vi "SendCommandToDeviceTCPWithRetry.vi"(6 "timeout ms":i32=100, 7 "ms to wait between retries":u32=50, 8 "error in":errorcluster, 9 "str command":string, 10 "connection refnum in":refnum<k5>, 11 "IP address":string) -> (0 "error out":errorcluster, 1 "str out":string, 2 "str to byte array":u8[](array[numeric]), 3 "connection refnum out":refnum<k5>)   [LabVIEW 2023]
doc: "Send a string command using a TCP connection.\nRetry multiple times until a connection is successful."
uses:
  GlobalVarsNetwork.vi
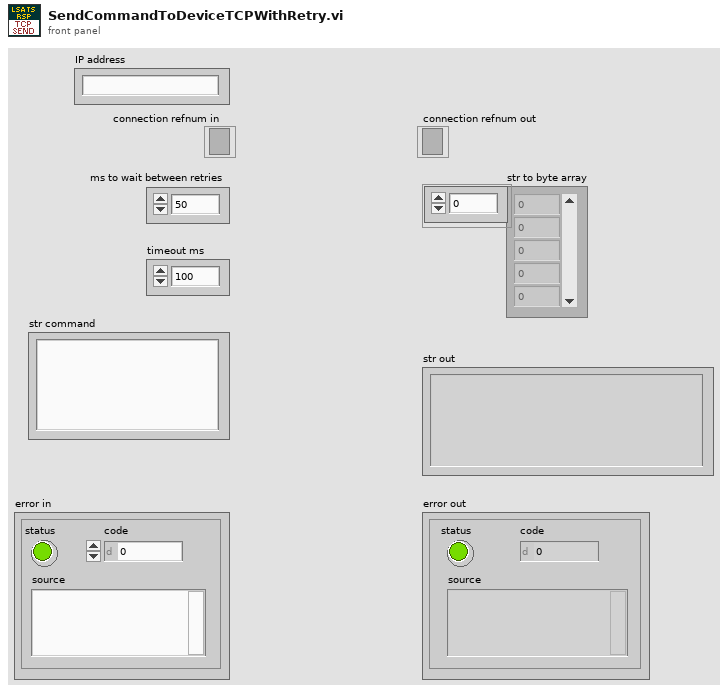
[diagram p1: front panel]
types:
  T1 = enum16{"Standard", "Buffered", "CRLF", "Immediate"}
  T2 = cluster{"XY_IP_ADDRESS":string, "Z_IP_ADDRESS":string, "Port":u16, "connection refnum x,y":refnum<k5>, "connection refnum z":refnum<k5>}
  T3 = enum16{"Initial Success", "Retry Successful", "Retry Failed"}
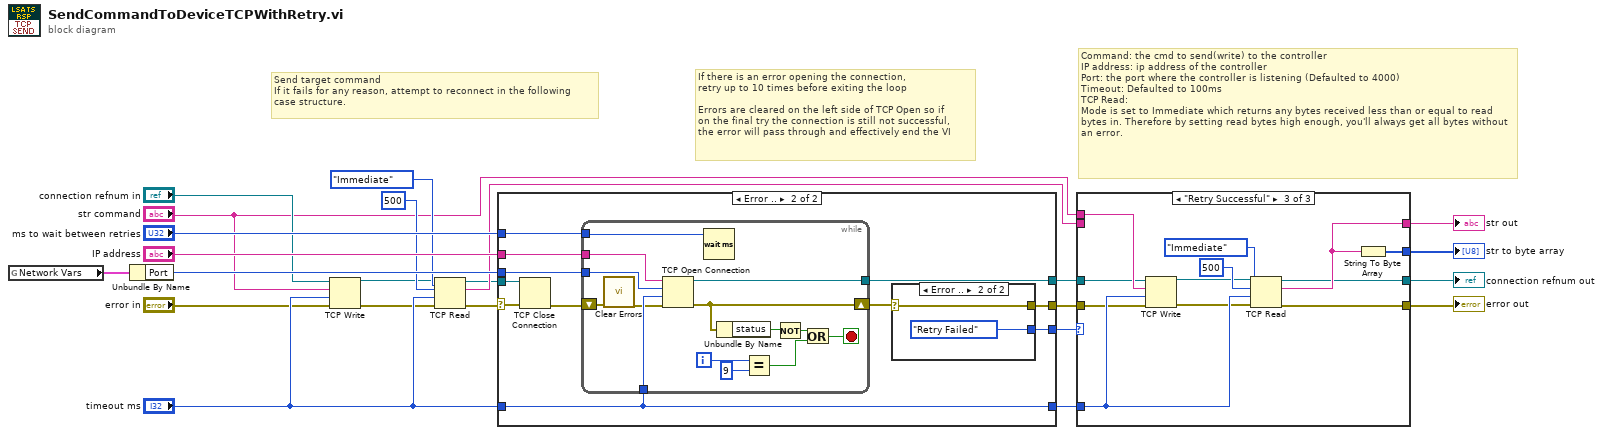
[diagram p0: block diagram]
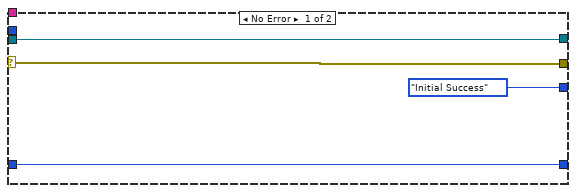
[diagram p2: hidden frame]
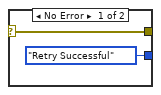
[diagram p3: hidden frame]
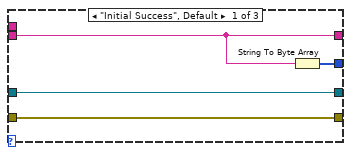
[diagram p4: hidden frame]
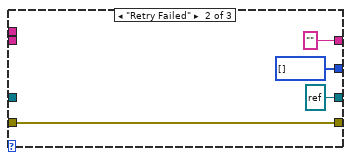
[diagram p5: hidden frame]
diagram:
  # "Send target command\nIf it fails for any reason, attempt to reconnect in the following\ncase structure."
  # "If there is an error opening the connection,\nretry up to 10 times before exiting the loop\n\nErrors are cleared on the left side of TCP Open so if \non the final try the connection is still not successful, \nthe error will pass through and effectively end the VI"
  # "Command: the cmd to send(write) to the controller\nIP address: ip address of the controller\nPort: the port where the controller is listening (Defaulted to 4000)\nTimeout: Defaulted to 100ms\nTCP Read:\nMode is set to Immediate which returns any bytes received less than or equal to read bytes in. Therefore by setting read bytes high enough, you'll always get all bytes without an error."
  n1 = global read "GlobalVarsNetwork.vi" "Network Vars"() -> (w20:T2)
  n2 = Unbundle By Name(w20) -> ("Port"=w19:u16)
  n3 = TCP Write(connection ID="connection refnum in", data in="str command", error in (no error)="error in", 9:"timeout ms") -> (connection ID out=w11:refnum<k5>, error out=w10:errorcluster)  [unwired: 1 out]
  n4 = TCP Read(connection ID=w11, bytes to read=500, error in (no error)=w10, 7:T1."Immediate" ("mode (standard)"), 9:"timeout ms") -> (connection ID out=w1:refnum<k5>, data out=w5:string, error out=w2:errorcluster)
  n5 = case shown="Error .." w2 {
    selector: w2 -> [w24 w29]
    tunnel: w19 -> [_ w38]
    tunnel: [w27 w37] -> w18
    tunnel: "ms to wait between retries" -> [_ w36]
    tunnel: "IP address" -> [_ w35]
    tunnel: "timeout ms" -> [w26 w34]
    tunnel: w1 -> [w27 w30]
    tunnel: [w26 w34] -> w7
    tunnel: [T3."Initial Success" w32] -> w4
    tunnel: [w24 w31] -> w3
    frame No Error {
    }
    frame Error {
      n6 = TCP Close Connection(connection ID=w30, error in (no error)=w29) -> (error out=w28:errorcluster)  [unwired: 1 in, 1 out]
      n7 = while {
        tunnel: w35 -> [w56]
        tunnel: w38 -> [w55]
        tunnel: [w54] -> w37
        tunnel: w34 -> [w47]
        shift-right: [w48] -> w33
        shift-left: w28 -> [w46]
        tunnel: w36 -> [w44]
        i -> [w53]
        stop <- w43 stop-if-true
        n8 = call <vilib>:"Clear Errors.vi"("error in (no error)"=w46) -> ("error out"=w45:errorcluster)  [unwired: 5 in, 1 out]
        n9 = TCP Open Connection(address=w56, remote port or service name=w55, timeout ms (60000)=w47, error in (no error)=w45) -> (connection ID=w54:refnum<k5>, error out=w48:errorcluster)  [unwired: 1 in]
        n10 = Wait (ms)(milliseconds to wait=w44) -> ()  [unwired: 1 out]
        n11 = Unbundle By Name(w48) -> ("status"=w50:bool)
        n12 = Equal?(x=w53, y=9) -> (x = y?=w51:bool)
        n13 = Not(x=w50) -> (.not. x?=w49:bool)
        n14 = Or(x=w49, y=w51) -> (x .or. y?=w43:bool)
      }
      n15 = case shown="Error .." w33 {
        selector: w33 -> [w39 w41]
        tunnel: [T3."Retry Successful" T3."Retry Failed"] -> w32
        tunnel: [w39 w41] -> w31
        frame No Error {
        }
        frame Error {
        }
      }
    }
  }
  n16 = case shown="\"Retry Successful\"" w4 {
    tunnel: [w57 w61 w65] -> w23
    tunnel: [w59 "" ("data out") w76] -> w22
    tunnel: [w60 u8[] [] ("unsigned byte array") w75] -> w21
    tunnel: w18 -> [w58 _ w68]
    tunnel: "str command" -> [_ _ w72]
    tunnel: w7 -> [_ _ w71]
    tunnel: [w58 refnum<k5> refnum ("connection ID") w66] -> w8
    tunnel: w5 -> [w59 _ _]
    tunnel: w3 -> [w57 w61 w67]
    frame "Initial Success", Default {
      n17 = String To Byte Array(string=w59) -> (unsigned byte array=w60:u8[])
    }
    frame "Retry Failed" {
    }
    frame "Retry Successful" {
      n18 = TCP Write(connection ID=w68, data in=w72, error in (no error)=w67, 9:w71) -> (connection ID out=w70:refnum<k5>, error out=w69:errorcluster)  [unwired: 1 out]
      n19 = TCP Read(connection ID=w70, bytes to read=500, error in (no error)=w69, 7:T1."Immediate" ("mode (standard)"), 9:w71) -> (connection ID out=w66:refnum<k5>, data out=w76:string, error out=w65:errorcluster)
      n20 = String To Byte Array(string=w76) -> (unsigned byte array=w75:u8[])
    }
  }
  "error out" <- w23
  "str to byte array" <- w21
  "str out" <- w22
  "connection refnum out" <- w8
